vi "Subvi counter U16.vi"(8 "Reset":bool, 9 "+1":bool) -> (1 "Count":u16)   [LabVIEW 2017]
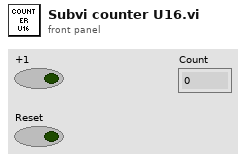
[diagram p1: front panel]
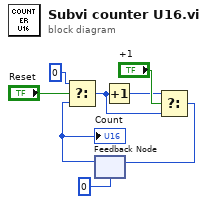
[diagram p0: block diagram]
diagram:
  n1 = feedback #1(u16 0) -> (w1:u16)
  "Count" <- w1
  n2 = Select(t=u16 0, s="Reset", f=w1) -> (s? t:f=w2:u16)
  n3 = Increment(x=w2) -> (x+1=w4:u16)
  n4 = Select(t=w4, s="+1", f=w2) -> (s? t:f=w7:u16)
  n5 = feedback-in #1(w7) -> ()
